vi "Delete User.vi"(3 "error in (no error)":errorcluster, 4 "UserID":i32, 5 "Database.lvlib:Data Store.lvclass":refnum<class "Data Store.lvclass">) -> (0 "error out":errorcluster, 2 "Database.lvlib:Data Store.lvclass 2":refnum<class "Data Store.lvclass">)   [LabVIEW 2011, in "Database.lvlib" / "Data Store.lvclass"]
uses:
  Data Store.lvclass
  Data Store.lvclass/Data Store.ctl
  <vilib>/addons/database/Connection.llb/Conn Execute.vi
  <vilib>/addons/database/Recordset.llb/Rec Destroy - Connection.vi
  <vilib>/addons/database/NI_Database_API.lvlib
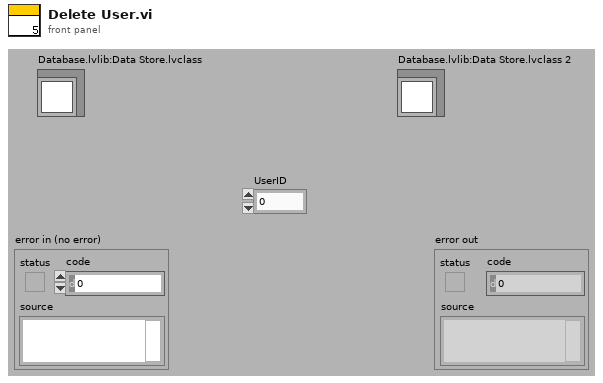
[diagram p1: front panel]
types:
  T1 = typedef "NI_Database_API.lvlib/Conn ObjectReference.ctl" = refnum<k1>
  T2 = typedef "NI_Database_API.lvlib/Rec ObjectReference.ctl" = refnum<k1>
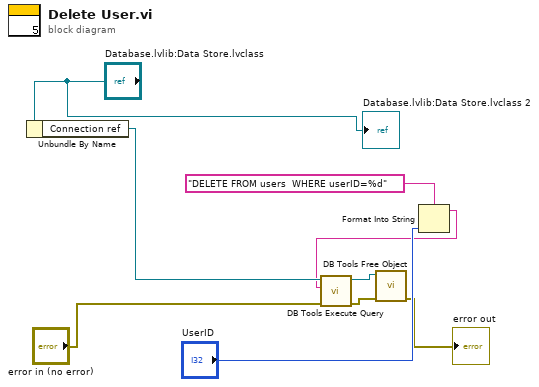
[diagram p0: block diagram]
diagram:
  n1 = Unbundle By Name("Database.lvlib:Data Store.lvclass") -> ("Connection ref"=w9:T1)
  n2 = Format Into String(format string="DELETE FROM users  WHERE userID=%d", "UserID") -> (resulting string=w6:string)  [unwired: 2 in, 1 out]
  n3 = call-poly <vilib>:"DB Tools Execute Query.vi"("error in (no error)"="error in (no error)", "SQL query"=w6, "connection reference"=w9) -> ("error out"=w2:errorcluster, "recordset reference"=w3:T2)  [unwired: 5 in]
  n4 = call-poly <vilib>:"DB Tools Free Object.vi"("error in (no error)"=w2, "recordset reference"=w3) -> ("error out"=→"error out":errorcluster)  [unwired: 8 in, 1 out]
  "Database.lvlib:Data Store.lvclass 2" <- "Database.lvlib:Data Store.lvclass"
